vi "Global Variable.vi"() -> ()   [LabVIEW 2020, in "Global Fixture Test Double.lvclass"]
uses:
  Global Fixture Test Double.lvclass
panel:
  out "Calls to Teardown":i32
  out "Calls to Setup":i32
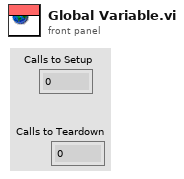
[diagram p1: front panel]
diagram:
